vi "Climb Controller.vi"(8 "error in":errorcluster) -> ()   [LabVIEW 2025]
doc: "This VI executes continuously carrying out the current operation and responding to updates or new operations. It will often contain the timing or control code that is difficult to place directly in TeleOp. This VI generally opens all sensors and motors and isolates the rest of the robot code from knowing how the operations are carried out."
uses:
  <vilib>/Rock Robotics/WPI/Framework/Completion Status.ctl
  Climb Setpoints.ctl
  Climb Operations.ctl
  <vilib>/Rock Robotics/WPI/ThirdParty/REV Robotics/REVLib/Typedef/SPARK PID Gains.ctl
  <vilib>/Rock Robotics/WPI/ThirdParty/REV Robotics/REVLib/Typedef/SPARK Feed Forward Gains.ctl
  <vilib>/Rock Robotics/WPI/ThirdParty/REV Robotics/REVLib/Typedef/Spark MAX Idle Mode.ctl
  <vilib>/Rock Robotics/WPI/ThirdParty/REV Robotics/REVLib/Typedef/Spark MAX Control Type.ctl
  <vilib>/Rock Robotics/WPI/ThirdParty/REV Robotics/REVLib/SubVI/Public/SPARK Open Brushless.vi
  <vilib>/Rock Robotics/WPI/ThirdParty/REV Robotics/REVLib/SubVI/Public/SPARK Configure Closed Loop Gains.vi
  <vilib>/Rock Robotics/WPI/ThirdParty/REV Robotics/REVLib/SubVI/Public/SPARK Configure Power Current Limit.vi
  <vilib>/Rock Robotics/WPI/ThirdParty/REV Robotics/REVLib/SubVI/Public/SPARK Configure Basic Idle Mode.vi
  <vilib>/Rock Robotics/Network Tables/NT Write Boolean.vi
panel:
  in  "Retracted Setpoint":dbl
  in  "Extended Setpoint":dbl
  in  "Climb  FF":T1
  in  "Climb PID":T2
  in  "Interactive Values":T3
  out "Current\nCmd":string
  in  "Buttons":cluster{"Execute Cmd":bool, "Abort Cmd":bool}
  out "Command Timing":cluster{"Start Time (ms)":u32, "Iterations":i32}
  out "Status":T5
  # "Interactive Command: You may fill in the settings for a command\nand schedule it with the Execute button. You can observe and abort\nany command while fine tuning the code for the controller."
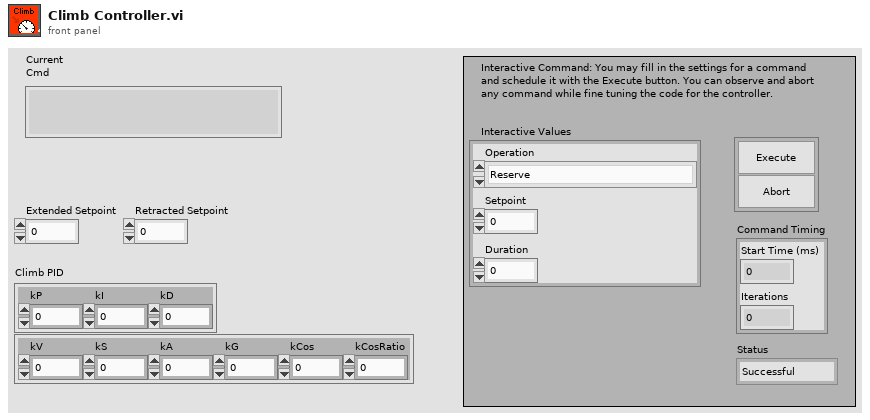
[diagram p1: front panel]
types:
  T1 = typedef "SPARK Feed Forward Gains.ctl" = cluster{"kV":dbl, "kS":dbl, "kA":dbl, "kG":dbl, "kCos":dbl, "kCosRatio":dbl}
  T2 = typedef "SPARK PID Gains.ctl" = cluster{"kP":dbl, "kI":dbl, "kD":dbl}
  T3 = typedef "Climb Setpoints.ctl" = cluster{"Operation":T4, "Setpoint":dbl, "Duration":dbl}
  T4 = typedef "Climb Operations.ctl" = enum16{"Reserve", "Read Current", "Retract Climb", "Extend Climb", "Immediate"}
  T5 = typedef "Completion Status.ctl" = enum16{"Successful", "Aborted", "Incomplete"}
  T6 = typedef "Spark MAX Idle Mode.ctl" = enum16{"Coast", "Brake"}
  T7 = typedef "WPI_MotorControlDeviceRef.ctl" = cluster{"DeviceStatus":errorcluster, "Type":T8, "PWM":cluster{"PWM Channel":T9, "DeadBand":T10}, "CAN":cluster{"Device Number":u8, "SetOutput VI Ref":variant, "GetOutput VI Ref":variant, "Enable VI Ref":variant, "Disable VI Ref":variant, "Data":variant}, "Invert":bool, "DIO PWM":cluster{"PWM \"Enable\" Channel":T9, "DIOChannel":T11, "PWM Rate":dbl}}
  T8 = typedef "WPI_MotorControlType.ctl" = enum16{"PWM", "CAN", "DIO PWM"}
  T9 = typedef "FPGA_DIOPWMChannel.ctl" = enum8{"PWM 0", "PWM 1", "PWM 2", "PWM 3", "PWM 4", "PWM 5", "PWM 6", "PWM 7", "PWM 8", "PWM 9", "PWM MXP 0", "PWM MXP 1", "PWM MXP 2", "PWM MXP 3", "PWM MXP 4", "PWM MXP 5", "PWM MXP 6", "PWM MXP 7", "PWM MXP 8", "PWM MXP 9", "Invalid"}
  T10 = typedef "WPI_PWMDeadband.ctl" = cluster{"Name":string, "maxPositivePwm":i32, "minPositivePwm":i32, "centerPwm":i32, "maxNegativePwm":i32, "minNegativePwm":i32, "angularRange":u16}
  T11 = typedef "FPGA_DIOChannel.ctl" = enum8{"DIO 0", "DIO 1", "DIO 2", "DIO 3", "DIO 4", "DIO 5", "DIO 6", "DIO 7", "DIO 8", "DIO 9", "DIO MXP 0", "DIO MXP 1", "DIO MXP 2", "DIO MXP 3", "DIO MXP 4", "DIO MXP 5", "DIO MXP 6", "DIO MXP 7", "DIO MXP 8", "DIO MXP 9", "DIO MXP 10", "DIO MXP 11", "DIO MXP 12", "DIO MXP 13", "DIO MXP 14", "DIO MXP 15", "SPI Port CS1", "SPI Port CS2", "SPI Port CS3", "SPI Port MISO", "SPI Port MOSI", "Invalid"}
  T12 = typedef "Command Status Info.ctl" = cluster{"Name":string, "Status":T5, "notifier out":T13}
  T13 = typedef "Completion Notifier.ctl" = refnum<notifier>
  T14 = cluster{"Current Command":T3, "Command Timing":cluster{"Start Time (ms)":u32, "Iterations":i32}, "Command Arguments":cluster{"Command Info":T12, "Description":string, "Default Command":T3, "queue out":refnum<queue>, "Subsystem Name":string}}
  T15 = typedef "Spark MAX Control Type.ctl" = enum16{"Percent VBus", "Voltage", "Velocity", "Position", "Smart Motion", "Current", "Smart Velocity", "MAXMotion Position", "MAXMotion Velocity"}
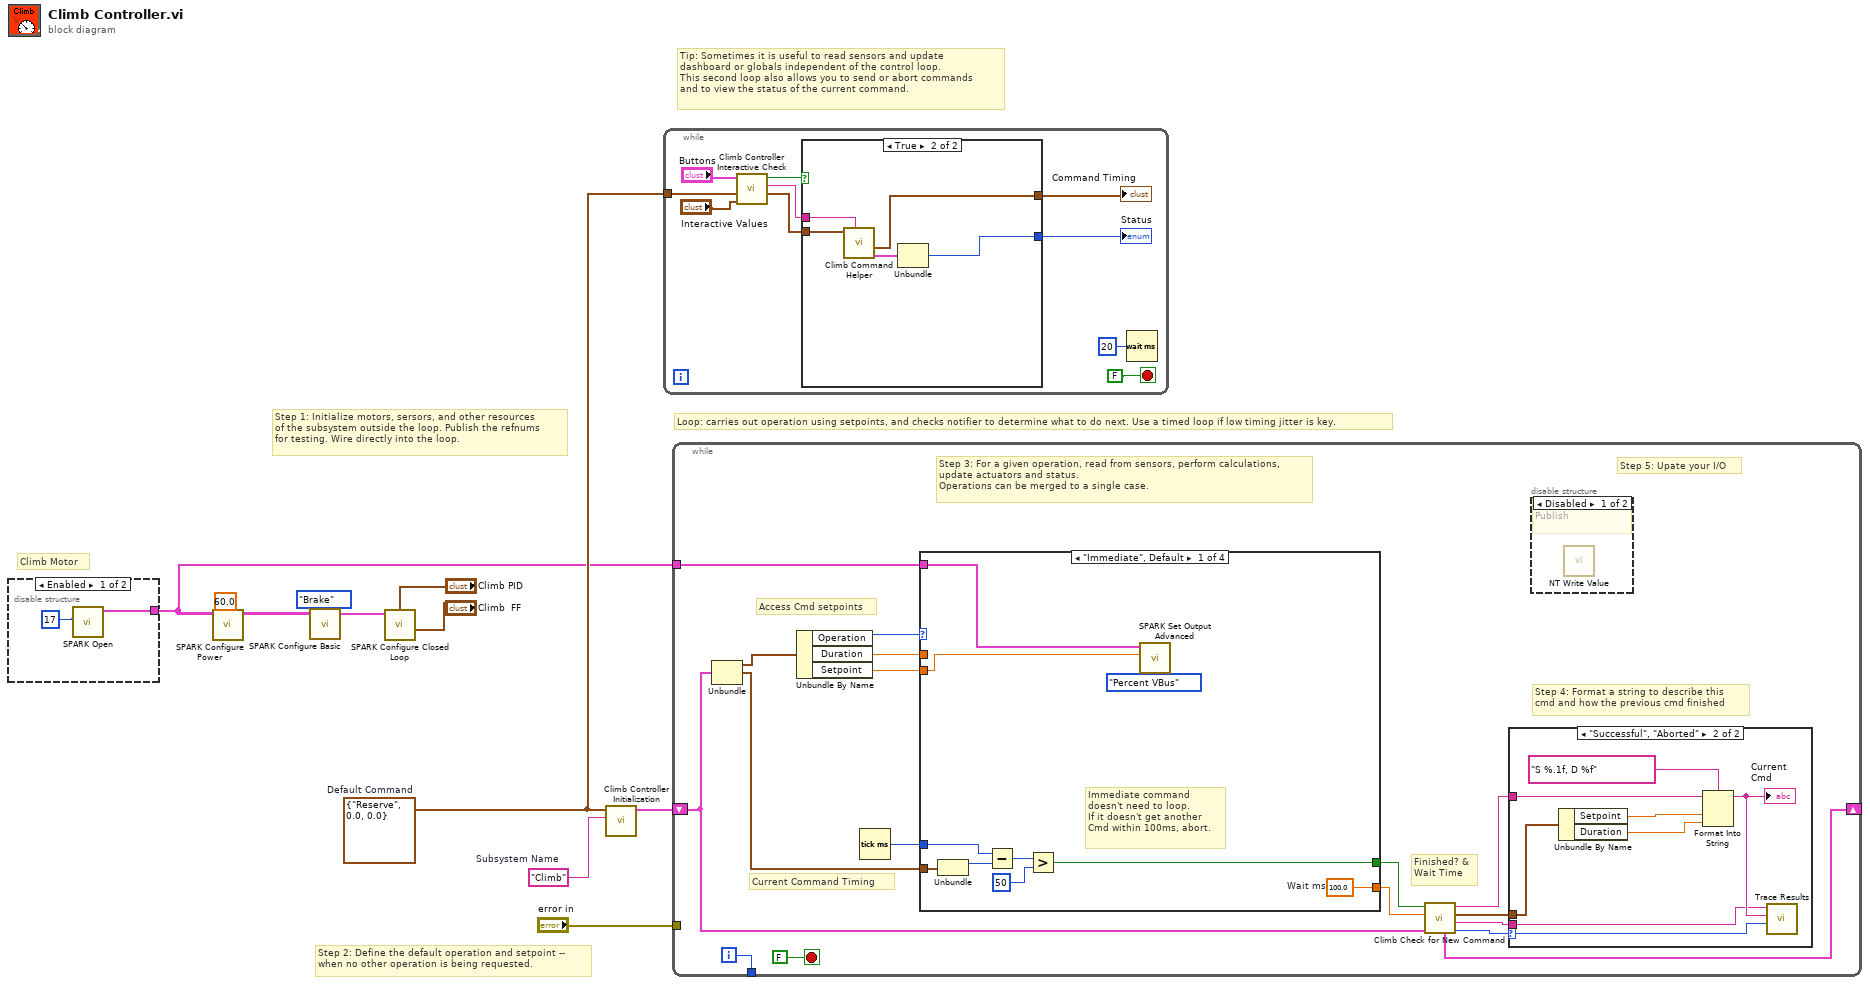
[diagram p0: block diagram]
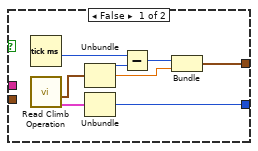
[diagram p3: hidden frame]
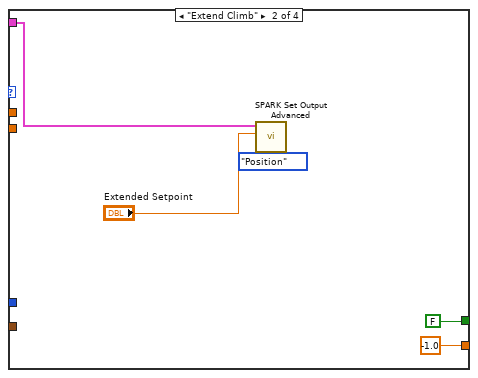
[diagram p6: hidden frame]
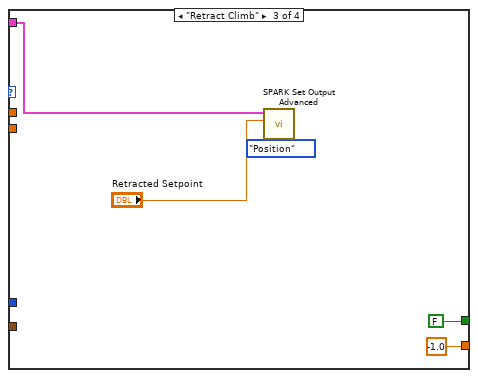
[diagram p7: hidden frame]
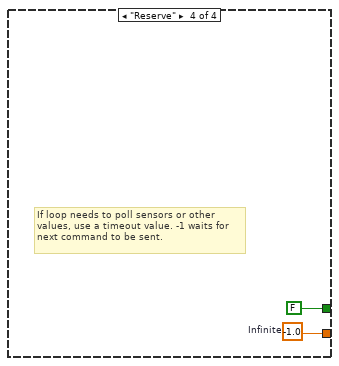
[diagram p8: hidden frame]
diagram:
  w6 = T3 {"Operation"=enum."Reserve", "Setpoint"=0.0, "Duration"=0.0}  # Default Command
  w7 = "Climb"  # Subsystem Name
  # "Climb Motor"
  # "Tip: Sometimes it is useful to read sensors and update\ndashboard or globals independent of the control loop.\nThis second loop also allows you to send or abort commands\nand to view the status of the current command."
  # "Step 2: Define the default operation and setpoint --\nwhen no other operation is being requested."
  # "Step 1: Initialize motors, sersors, and other resources\nof the subsystem outside the loop. Publish the refnums\nfor testing. Wire directly into the loop."
  # "Loop: carries out operation using setpoints, and checks notifier to determine what to do next. Use a timed loop if low timing jitter is key."
  n1 = disable-structure shown="Enabled" {
    disable-tunnel: [w10 _] -> w1
    frame Enabled {
      n2 = call-poly <vilib>:"SPARK Open.vi"("Device Number"=u8 17) -> ("MotorControlDeviceRef"=w10:T7)  [unwired: 9 in, 1 out]
    }
    frame Disabled {
    }
  }
  n3 = call-poly <vilib>:"SPARK Configure Power.vi"("Current Limit A (100)"=sgl 60.0, "MotorControlDeviceRef in"=w1) -> ()  [unwired: 8 in, 2 out]
  n4 = call-poly <vilib>:"SPARK Configure Basic.vi"("Idle Mode"=Spark_MAX_Idle_Mode."Brake", "MotorControlDeviceRef in"=w1) -> ()  [unwired: 8 in, 2 out]
  n5 = call-poly <vilib>:"SPARK Configure Closed Loop.vi"("Feed Forward Gains"="Climb  FF", "PID Gains"="Climb PID", "MotorControlDeviceRef in"=w1) -> ()  [unwired: 7 in, 2 out]
  n6 = call "Climb Controller Initialization.vi"("Subsystem Name"=w7, "Default Command"=w6) -> ("Current Command"=w8:T14)  [unwired: 9 in]
  n7 = while {
    tunnel: w6 -> [w18]
    stop <- FALSE stop-if-true
    n8 = call "Climb Controller Interactive Check.vi"("Interactive Command in"="Interactive Values", "Default Command"=w18, "Buttons"="Buttons") -> ("Interactive Command out"=w15:T3, "Trace String"=w16:string, "Schedule"=w17:bool)  [unwired: 6 in]
    n9 = case shown="True" w17 {
      tunnel: [w29 w34] -> w14
      tunnel: w15 -> [_ w32]
      tunnel: [w25 w30] -> w13
      tunnel: w16 -> [_ w33]
      frame False {
        n10 = Tick Count (ms)() -> (millisecond timer value=w24:u32)
        n11 = call "Read Climb Operation.vi"() -> ("Command Info"=w22:T12, "SubSystem Data"=w23:T3)  [unwired: 9 in, 1 out]
        n12 = Unbundle(w23) -> ("Operation"=w28:T4, "Setpoint"=w26:dbl)  [unwired: 1 out]
        n13 = Unbundle(w22) -> ("Status"=w29:T5)  [unwired: 2 out]
        n14 = Subtract(x=w24, y=w28) -> (x-y=w27:u32)
        n15 = Bundle(w27, "Setpoint"=w26) -> (w25:cluster{u32, "Setpoint":dbl})  [unwired: 1 in]
      }
      frame True {
        n16 = call "Climb Command Helper.vi"("Description"=w33, "SubSystem Data"=w32) -> ("Command Info Out"=w31:T12, "Command Timing"=w30:cluster{"Start Time (ms)":u32, "Iterations":i32})  [unwired: 7 in, 1 out]
        n17 = Unbundle(w31) -> ("Status"=w34:T5)  [unwired: 2 out]
      }
    }
    "Status" <- w14
    "Command Timing" <- w13
    n18 = Wait (ms)(milliseconds to wait=u32 20) -> ()  [unwired: 1 out]
  }
  n19 = while {
    shift-right: [w43] -> _
    shift-left: w8 -> [w36]
    tunnel: [w50] -> _
    tunnel: "error in" -> [_]
    tunnel: w1 -> [w35]
    i -> [w50]
    stop <- FALSE stop-if-true
    # "Step 5: Upate your I/O"
    # "Step 4: Format a string to describe this\ncmd and how the previous cmd finished"
    # "Current Command Timing"
    # "Access Cmd setpoints"
    # "Finished? &\nWait Time"
    # "Step 3: For a given operation, read from sensors, perform calculations,\nupdate actuators and status.\nOperations can be merged to a single case."
    n20 = Unbundle(w36) -> ("Current Command"=w49:T3, "Command Timing"=w45:cluster{"Start Time (ms)":u32, "Iterations":i32})  [unwired: 1 out]
    n21 = Unbundle By Name(w49) -> ("Operation"=w48:T4, "Duration"=w47:dbl, "Setpoint"=w44:dbl)
    n22 = Tick Count (ms)() -> (millisecond timer value=w46:u32)
    n23 = case shown="\"Immediate\", Default" w48 {
      tunnel: [w69 -1.0 ("Infinite") -1.0 ("Infinite") w81] -> w41
      tunnel: [w63 FALSE ("ignore previous (F)") FALSE ("ignore previous (F)") FALSE ("ignore previous (F)")] -> w42
      tunnel: w45 -> [w65 _ _ _]
      tunnel: w47 -> [_ _ _ _]
      tunnel: w46 -> [w64 _ _ _]
      tunnel: w44 -> [w60 _ _ _]
      tunnel: w35 -> [w61 w70 w75 _]
      frame "Immediate", Default {
        w69 = 100.0  # Wait ms
        # "Immediate command\ndoesn't need to loop.\nIf it doesn't get another\nCmd within 100ms, abort."
        n24 = Unbundle(w65) -> ("Start Time (ms)"=w68:u32)  [unwired: 1 out]
        n25 = Subtract(x=w64, y=w68) -> (x-y=w67:u32)
        n26 = Greater?(x=w67, y=u8 50 ("Left Motor")) -> (0:w63:bool)
        n27 = call <vilib>:"SPARK Set Output Advanced.vi"("Control Mode"=Spark_MAX_Control_Type."Percent VBus", "Setpoint"=w60, "MotorControlDevRef"=w61) -> ()  [unwired: 7 in, 2 out]
      }
      frame "Extend Climb" {
        n28 = call <vilib>:"SPARK Set Output Advanced.vi"("Control Mode"=Spark_MAX_Control_Type."Position", "Setpoint"="Extended Setpoint", "MotorControlDevRef"=w70) -> ()  [unwired: 7 in, 2 out]
      }
      frame "Retract Climb" {
        n29 = call <vilib>:"SPARK Set Output Advanced.vi"("Control Mode"=Spark_MAX_Control_Type."Position", "Setpoint"="Retracted Setpoint", "MotorControlDevRef"=w75) -> ()  [unwired: 7 in, 2 out]
      }
      frame "Reserve" {
        w81 = -1.0  # Infinite
        # "If loop needs to poll sensors or other\nvalues, use a timeout value. -1 waits for\nnext command to be sent."
      }
    }
    n30 = call "Climb Check for New Command.vi"("Current Command"=w36, "Wait time (ms)"=w41, "Finished?"=w42) -> ("Completion"=w37:T5, "Subsystem Name"=w38:string, "Current Command"=w39:T3, "Initial Trace String"=w40:string, "NextCommand"=w43:T14)  [unwired: 4 in]
    n31 = case shown="\"Successful\", \"Aborted\"" w37 {
      selector: w37 -> [_ w59]
      tunnel: w40 -> [_ w55]
      tunnel: w39 -> [_ w56]
      tunnel: w38 -> [_ w52]
      frame "Incomplete", Default {
        # "Continuing current command"
      }
      frame "Successful", "Aborted" {
        # "Report and setup for next command"
        n32 = Unbundle By Name(w56) -> ("Setpoint"=w58:dbl, "Duration"=w53:dbl)
        n33 = Format Into String(format string="S %.1f, D %f", initial string=w55, w58, w53) -> (resulting string=w54:string)  [unwired: 1 in, 1 out]
        "Current\nCmd" <- w54
        n34 = call <vilib>:"Trace Results.vi"("Status of previous command"=w59, "Description"=w54, "Subsystem"=w52) -> ()  [unwired: 9 in]
      }
    }
    n35 = disable-structure shown="Disabled" {
      frame Disabled {
        # "Publish"
        n36 = call-poly <vilib>:"NT Write Value.vi"() -> ()  [unwired: 11 in, 1 out]
      }
      frame Enabled {
      }
    }
  }
